vi "PH_HamamatsuCamera.panel.vi"(0 "object ref":refnum<vi>, 5 "error in (no error)":errorcluster) -> (19 "error out":errorcluster)   [LabVIEW 2014, in "PH_HamamatsuCamera.lvlib"]
doc: "This VI is the GUI to control a IEEE1394 Cam.\n\nLicense Agreement for this software:\n\nCopyright (C)\nGesellschaft für Schwerionenforschung, GSI\nPlanckstr. 1\n64291 Darmstadt\nGermany\n\nContact: D.Beck@gsi.de \n\nThis program is free software; you can redistribute it and/or modify it under the terms of the GNU General Public License as published by the Free Software Foundation; either version 2 of the license, or (at your option) any later version.\n\nThis program is distributed in the hope that it will be useful, but WITHOUT ANYW ARRANTY; without even the implied warranty of MERCHANTABILITY or FITNESS FOR A PARTICULAR PURPOSE. See the GNU General License for more details (http://www.gnu.org).\n\nGesellschaft für Schwerionenforschung, GSI\nPlanckstr. 1, 64291 Darmstadt, Germany\nFor all questions and ideas contact: M.Richter@gsi.de, H.Brand@gsi.de or D.Beck@gsi.de.\nLast update: 18-DEC-2002"
uses:
  PH_HamamatsuCamera.lvlib
  PH_StatusHandler/PH_StatusHandler.GUI element.ctl
  PH_HamamatsuCamera.ROI.ctl
  PH_HamamatsuCamera.Trigger Parameter.ctl
  PH_HamamatsuCamera.Parameter Set.ctl
  PH_HamamatsuCamera.Cam Parameter.ctl
  PH_Cam_BaseClass/PH_Cam_BaseClass.GUI Refs.ctl
  CSCore/CSObj/CSObj.lvlib
  CSCore/CSSystem/CSSystemLib/CSSystemLib.lvlib
  PH_Common/PH_Common.lvlib
  PH_Cam_BaseClass/PH_Cam_BaseClass.lvlib
  PH_Class/PH_Class.lvlib
  PH_StatusHandler/PH_StatusHandler.lvlib
panel:
  in  "Driver Original Polarity":u32(ring)=1 items=["Negative"=1, "Positive"=2]
  in  "Driver Original Mode":u32(ring)=1 items=["Internal"=1, "External Edge"=2, "External Level"=4, "Software"=32, "Fast Repetition"=64, "TDI"=128, "Trigger Start"=512, "Sync Readout"=1024]
  out "PSDB Status":u32(colorbox)=6618880 caption="PSDB"
  out "Status":T1 caption="Camera"
  in  "Tab Control":T2(tab)
  in  "Trigger Timeout":u32=1000 caption="ms"
  in  "Gain":dbl
  in  "Brightness":dbl
  in  "Shutter":dbl caption="s"
  in  "Start Cam":bool
  in  "Get Histogram":bool
  in  "Logarithmic":bool
  out "Histogram":u32[](graph)
  in  "Trigger Polarity":u32(ring) items=["No Info"]
  in  "Trigger Mode":u32(ring) items=["No Info"]
  in  "Save Image":bool
  in  "Show Image":bool
  in  "Palette":i32(ring) items=["Grey", "Binary", "Gradient", "Rainbow", "Temperature", "HMH"]
  in  "Scale Factor":i32=50 caption="%" min=30 max=500
  in  "Center of Gravity":bool
  in  "Subtract Background":bool
  in  "Center Cross":bool
  in  "Set ROI to Maximum":bool
  in  "ROI":T3
  out "Camera Details":T4
  out "Cam Error":errorcluster
  in  "Cam List":u32(ring)
  out "Frames per second":dbl(knob) scale=0.0..30.0 scale format="%.1f"
  in  "Get Frame Rate":bool
  in  "Parameter to set":T5=4212128 items=["SENSOR MODE"=4212128, "CCD MODE"=4212384, "READOUT MODE"=4211872, "ACTIVE VIEW INDEX"=4343136, "BITS PER CHANNEL"=4342976, "IMAGE PIXEL TYPE"=4343296, "BINNING"=4215968, "EXPOSURE TIME"=2049184, "CONTRAST GAIN"=3163312, "CONTRAST OFFSET"=3163328, "LIGHT MODE"=2114720, "SENSITIVITY"=2114992, "PHOTON IMAGING MODE"=2115200, "HIGH DYNAMIC RANGE MODE"=3163360, "WHITE BALANCE"=3163568, "TEMPERATURE"=2115232, "TEMPERATURE TARGET"=2115264, "SENSOR COOLER FAN"=2115296, "LINEBUNDLE HEIGHT"=4212192, "MECHANICAL SHUTTER"=2115488, "BACK FOCUS POSITION"=8422304, "TRIGGER CONNECTOR"=1066432, "TRIGGER SOURCE"=1066144, "OUTPUT TRIGGER SOURCE"=1852576, "TRIGGER GLOBAL EXPOSURE"=2049680, "FIRST TRIGGER BEHAVIOR"=2049696, "CHANNEL SYNC"=1852352, "READOUT DIRECTION"=4211904, "PRE HSYNC COUNT"=1852704, "INTERNAL LINE SPEED"=4191408, "INTERNAL LINE INTERVAL"=4191424]
  in  "Set Cam Parameter":bool caption="Set"
  in  "Value to set":dbl caption="Value"
  out "Parameters":T6[](array[typedef])
  in  "Trigger Parameters":T7={"Mode"=1, "Polarity"=1, "Times"=1, "Delay"=0.0} {"Polarity" items=["Negative"=1, "Positive"=2]; "Mode" items=["Internal"=1, "External Edge"=2, "External Level"=4, "Software"=32, "Fast Repetition"=64, "TDI"=128, "Trigger Start"=512, "Sync Readout"=1024]}
  in  "Delete":bool
  in  "Exit":bool
  # "PCS"
  # "3.40"
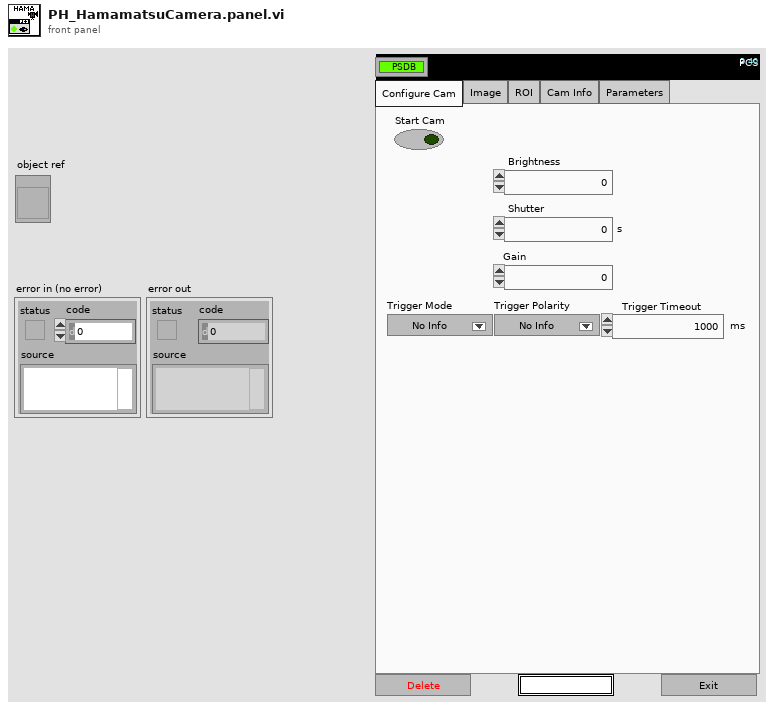
[diagram p1: front panel]
types:
  T1 = typedef "PH_StatusHandler.lvlib/PH_StatusHandler.GUI element.ctl" = u16
  T2 = enum32{"Configure Cam", "Image", "ROI", "Cam Info", "Parameters"}
  T3 = typedef "PH_HamamatsuCamera.lvlib/PH_HamamatsuCamera.ROI.ctl" = cluster{"Horizontal Offset":i32, "Vertical Offset":i32, "Horizontal Width":i32, "Vertical Width":i32}
  T4 = cluster{"Model":string, "Camera ID":string, "Firmware":string}
  T5 = typedef "PH_HamamatsuCamera.lvlib/PH_HamamatsuCamera.Cam Parameter.ctl" = u32
  T6 = typedef "PH_HamamatsuCamera.lvlib/PH_HamamatsuCamera.Parameter Set.ctl" = cluster{"Parameter":string, "Value":dbl, "Writable":bool, "Range":cluster{"min":dbl, "max":dbl, "step":dbl}, "Default":dbl, "Value Names":cluster{"Name":string, "Value":dbl}[], "Text Values":bool}
  T7 = typedef "PH_HamamatsuCamera.lvlib/PH_HamamatsuCamera.Trigger Parameter.ctl" = cluster{"Mode":u32, "Polarity":u32, "Times":u32, "Delay":dbl}
  T8 = typedef "PH_Cam_BaseClass.lvlib/PH_Cam_BaseClass.GUI Refs.ctl" = cluster{"Frame Rate":refnum<vi>, "Get Frame Rate":refnum<vi>, "Show Image":refnum<vi>, "Get Histogram":refnum<vi>, "Mapping":refnum<vi>, "Histogram":refnum<vi>, "Center Cross":refnum<vi>, "Center of Gravity":refnum<vi>, "Scale Factor [%]":refnum<vi>, "Save Image":refnum<vi>, "Palette":refnum<vi>, "Subtract Background":refnum<vi>, "Cam Error":refnum<vi>, "On":refnum<vi>, "Cam List":refnum<vi>}
  T9 = cluster{"Cam Base ClassGui Refs":T8, "PSDB Status":refnum<vi>, "Status":refnum<vi>}
  T10 = typedef "PH_HamamatsuCamera.lvlib/PH_HamamatsuCamera.i attribute.ctl" = cluster{"Gui Refs":cluster{"Camera Details":refnum<vi>, "ROI":refnum<vi>, "Set ROI to Maximum":refnum<vi>, "Trigger Parameters":refnum<vi>, "Brightness":refnum<vi>, "Shutter":refnum<vi>, "Gain":refnum<vi>, "Trigger Timeout":refnum<vi>, "Trigger Polarity":refnum<vi>, "Trigger Mode":refnum<vi>, "Parameters":refnum<vi>, "Set Cam Parameter":refnum<vi>, "Parameter to set":refnum<vi>, "Value to set":refnum<vi>}, "Cam":cluster{"Handle":i32, "Details":cluster{"Model":string, "Camera ID":string, "Firmware":string}, "Buffer Info":cluster{"height":u32, "width":u32, "datatype":u32}}, "H Offset":cluster{"Value":i32, "Minimum":i32, "Maximum":i32, "Increment":i32}, "V Offset":cluster{"Value":i32, "Minimum":i32, "Maximum":i32, "Increment":i32}, "H Width":cluster{"Value":i32, "Minimum":i32, "Maximum":i32, "Increment":i32}, "V Width":cluster{"Value":i32, "Minimum":i32, "Maximum":i32, "Increment":i32}, "Trigger Parameters":T7, "Trigger Timeout":u32, "Parameters":T6[], "Indicees Cam Parameters":cluster{"Brightness":i32, "Shutter":i32, "Gain":i32}, "Wanted Values":cluster{"Trigger Settings":T7[], "ROI":T3[], "Parameter":cluster{"Name":string, "Value":dbl}[]}}
  T11 = typedef "LVStringsAndValuesArrayTypeDef_U32.ctl" = cluster{"String":string, "Value":u32}[]
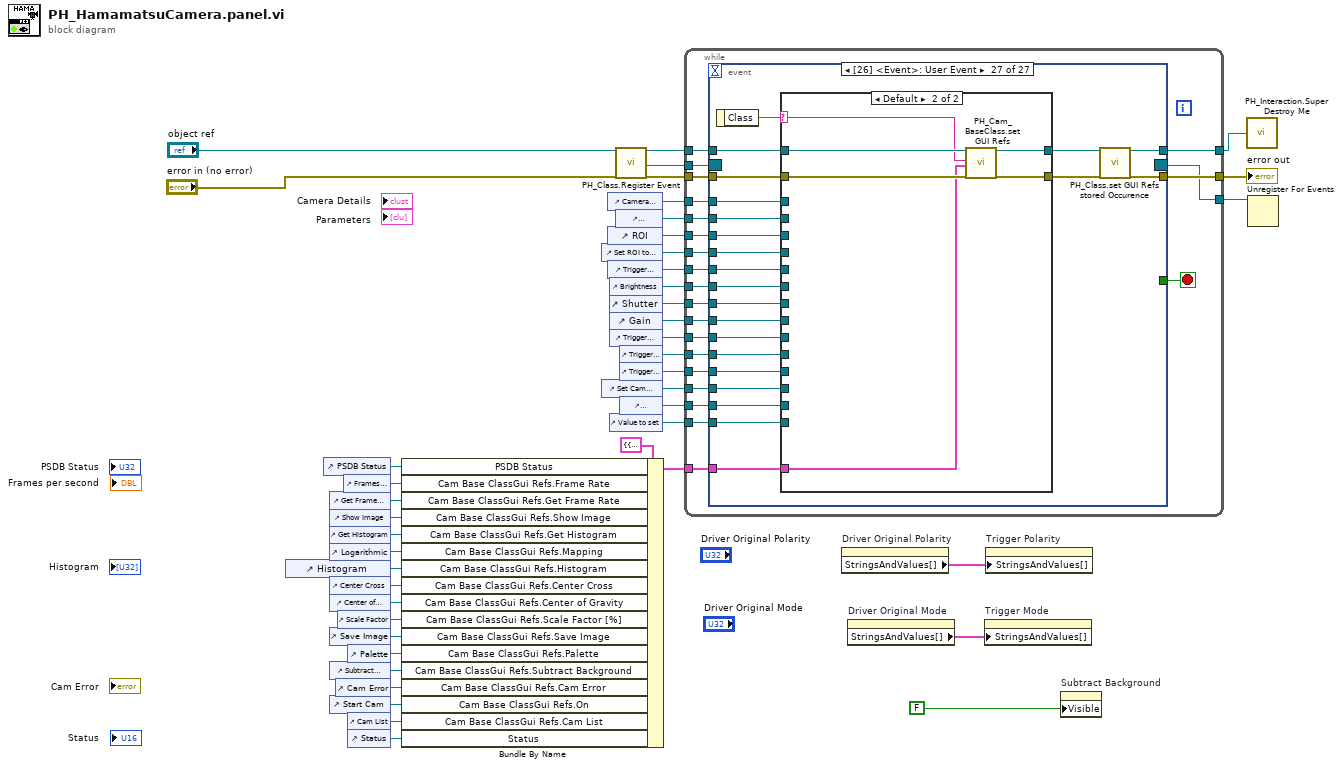
[diagram p0: block diagram]
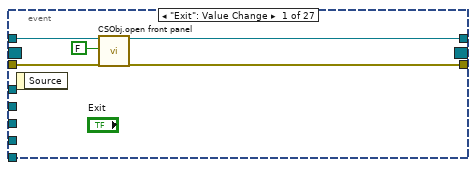
[diagram p2: hidden frame]
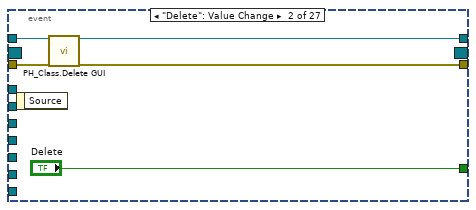
[diagram p3: hidden frame]
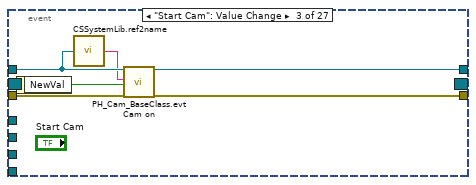
[diagram p4: hidden frame]
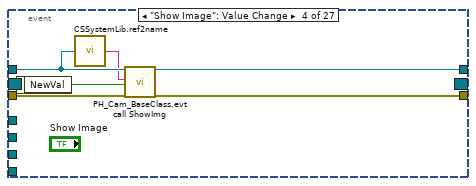
[diagram p5: hidden frame]
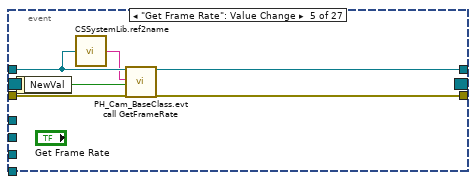
[diagram p6: hidden frame]
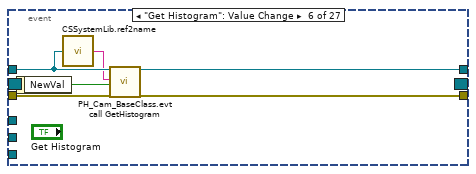
[diagram p7: hidden frame]
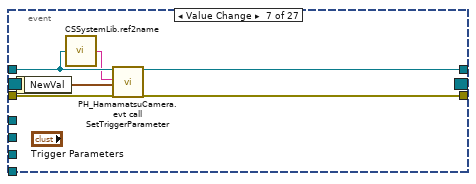
[diagram p8: hidden frame]
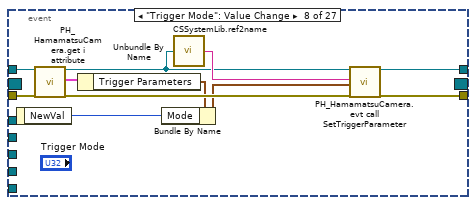
[diagram p9: hidden frame]
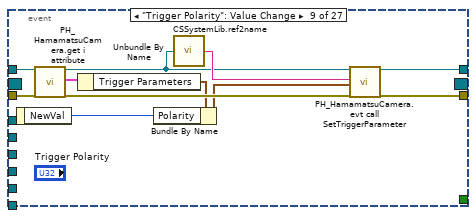
[diagram p10: hidden frame]
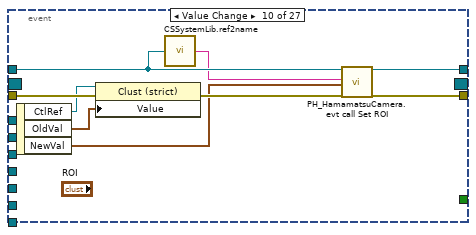
[diagram p11: hidden frame]
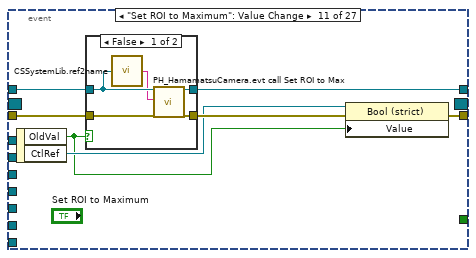
[diagram p12: hidden frame]
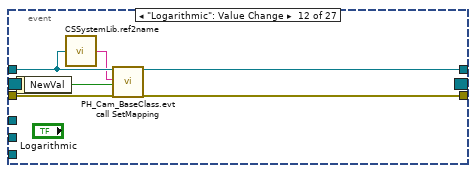
[diagram p14: hidden frame]
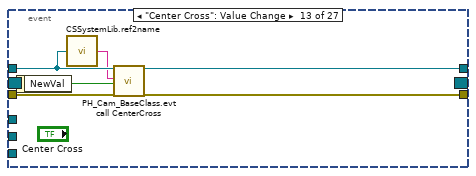
[diagram p15: hidden frame]
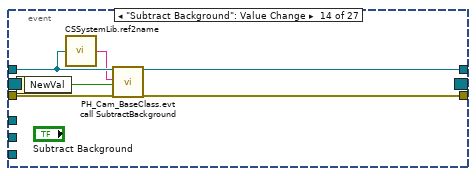
[diagram p16: hidden frame]
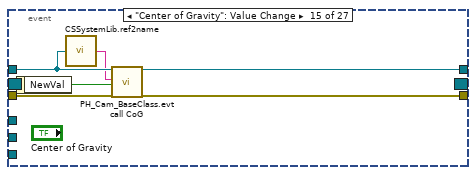
[diagram p17: hidden frame]
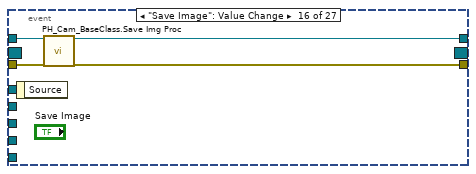
[diagram p18: hidden frame]
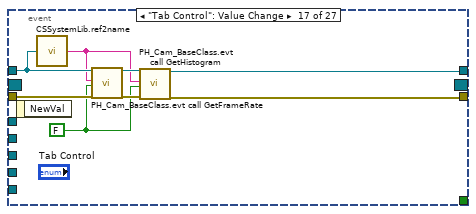
[diagram p19: hidden frame]
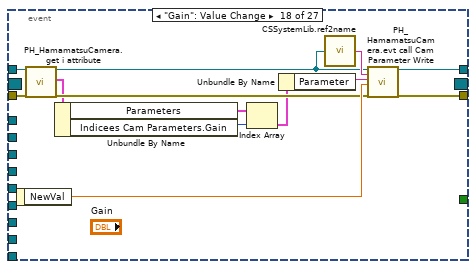
[diagram p20: hidden frame]
diagram:
  n1 = control-ref of="Histogram"() -> (w35:refnum<vi>)
  n2 = control-ref of="PSDB Status"() -> (w20:refnum<vi>)
  n3 = control-ref of="Get Frame Rate"() -> (w39:refnum<vi>)
  n4 = control-ref of="Show Image"() -> (w38:refnum<vi>)
  n5 = control-ref of="Get Histogram"() -> (w37:refnum<vi>)
  n6 = control-ref of="Logarithmic"() -> (w36:refnum<vi>)
  n7 = control-ref of="Center Cross"() -> (w34:refnum<vi>)
  n8 = control-ref of="Center of Gravity"() -> (w33:refnum<vi>)
  n9 = control-ref of="Save Image"() -> (w31:refnum<vi>)
  n10 = control-ref of="Subtract Background"() -> (w29:refnum<vi>)
  n11 = control-ref of="Start Cam"() -> (w26:refnum<vi>)
  n12 = control-ref of="Cam Error"() -> (w27:refnum<vi>)
  n13 = control-ref of="Scale Factor"() -> (w32:refnum<vi>)
  n14 = control-ref of="Frames per second"() -> (w40:refnum<vi>)
  n15 = control-ref of="Palette"() -> (w30:refnum<vi>)
  n16 = control-ref of="Cam List"() -> (w25:refnum<vi>)
  n17 = control-ref of="Status"() -> (w1:refnum<vi>)
  n18 = Bundle By Name(cluster=T9 {"Cam Base ClassGui Refs"={"Frame Rate"=refnum, "Get Frame Rate"=refnum, "Show Image"=refnum, "Get Histogram"=refnum, "Mapping"=refnum, "Histogram"=refnum, "Center Cross"=refnum, "Center of Gravity"=refnum, "Scale Factor [%]"=refnum, "Save Image"=refnum, "Palette"=refnum, "Subtract Background"=refnum, "Cam Error"=refnum, "On"=refnum, "Cam List"=refnum}, "PSDB Status"=refnum, "Status"=refnum} ("GUI Refs to set"), "PSDB Status"=w20, "Cam Base ClassGui Refs.Frame Rate"=w40, "Cam Base ClassGui Refs.Get Frame Rate"=w39, "Cam Base ClassGui Refs.Show Image"=w38, "Cam Base ClassGui Refs.Get Histogram"=w37, "Cam Base ClassGui Refs.Mapping"=w36, "Cam Base ClassGui Refs.Histogram"=w35, "Cam Base ClassGui Refs.Center Cross"=w34, "Cam Base ClassGui Refs.Center of Gravity"=w33, "Cam Base ClassGui Refs.Scale Factor [%]"=w32, "Cam Base ClassGui Refs.Save Image"=w31, "Cam Base ClassGui Refs.Palette"=w30, "Cam Base ClassGui Refs.Subtract Background"=w29, "Cam Base ClassGui Refs.Cam Error"=w27, "Cam Base ClassGui Refs.On"=w26, "Cam Base ClassGui Refs.Cam List"=w25, "Status"=w1) -> (w19:T9)
  n19 = control-ref of="Set ROI to Maximum"() -> (w15:refnum<vi>)
  n20 = control-ref of="Set Cam Parameter"() -> (w7:refnum<vi>)
  n21 = control-ref of="Camera Details"() -> (w18:refnum<vi>)
  n22 = control-ref of="ROI"() -> (w16:refnum<vi>)
  n23 = control-ref of="Trigger Parameters"() -> (w14:refnum<vi>)
  n24 = control-ref of="Brightness"() -> (w13:refnum<vi>)
  n25 = control-ref of="Shutter"() -> (w12:refnum<vi>)
  n26 = control-ref of="Gain"() -> (w11:refnum<vi>)
  n27 = control-ref of="Trigger Timeout"() -> (w10:refnum<vi>)
  n28 = control-ref of="Value to set"() -> (w5:refnum<vi>)
  n29 = call "PH_Class.Register Event.vi"("i ref in"="object ref", "error in (no error)"="error in (no error)") -> ("i ref out"=w24:refnum<vi>, "Event Registration Refnum"=w22:refnum<event-registration>, "error out"=w23:errorcluster)  [unwired: 15 in]
  n30 = control-ref of="Parameters"() -> (w17:refnum<vi>)
  n31 = control-ref of="Trigger Polarity"() -> (w9:refnum<vi>)
  n32 = control-ref of="Trigger Mode"() -> (w8:refnum<vi>)
  n33 = control-ref of="Parameter to set"() -> (w6:refnum<vi>)
  n34 = while {
    tunnel: w24 -> [w63]
    tunnel: [w62] -> w43
    tunnel: w23 -> [w65]
    tunnel: [w64] -> w44
    tunnel: w22 -> [w61]
    tunnel: [w60] -> w21
    tunnel: w19 -> [w59]
    tunnel: w18 -> [w58]
    tunnel: w17 -> [w57]
    tunnel: w16 -> [w56]
    tunnel: w15 -> [w55]
    tunnel: w14 -> [w54]
    tunnel: w13 -> [w53]
    tunnel: w12 -> [w52]
    tunnel: w11 -> [w51]
    tunnel: w10 -> [w50]
    tunnel: w9 -> [w49]
    tunnel: w8 -> [w48]
    tunnel: w7 -> [w47]
    tunnel: w6 -> [w46]
    tunnel: w5 -> [w45]
    stop <- w66 stop-if-true
    n35 = event shown="[26] <Event>: User Event" {
      selector: w61 -> [_ _ _ _ _ _ _ _ _ _ _ _ _ _ _ _ _ _ _ _ _ _ _ _ _ _ _]
      dyn-events: [_ _ _ _ _ _ _ _ _ _ _ _ _ _ _ _ _ _ _ _ _ _ _ _ _ _ _] -> w60
      timeout: _ -> [_ _ _ _ _ _ _ _ _ _ _ _ _ _ _ _ _ _ _ _ _ _ _ _ _ _ _]
      tunnel: [_ "Delete" _ _ _ _ _ _ _ _ _ _ _ _ _ _ _ _ _ _ _ _ _ _ _ _ _] -> w66
      tunnel: w63 -> [w71 w74 w79 w85 w91 w97 w103 w112 w123 w135 w141 w154 w160 w166 w172 w178 w182 w194 w207 w220 w229 w235 w243 w254 w264 w269 w293]
      tunnel: w65 -> [w69 w75 w82 w88 w94 w100 w106 w117 w128 w131 w144 w157 w163 w169 w175 w179 w185 w200 w213 w226 w232 w238 w246 w248 w262 w271 w292]
      tunnel: [w68 w72 w81 w87 w93 w99 w105 w116 w127 w137 w140 w156 w162 w168 w174 w176 w183 w198 w211 w224 w230 w236 w244 w255 w265 w270 w287] -> w64
      tunnel: [w67 w73 w80 w86 w92 w98 w104 w115 w126 w136 w142 w155 w161 w167 w173 w177 w186 w199 w212 w225 w231 w237 w245 w256 w266 w268 w289] -> w62
      tunnel: w59 -> [_ _ _ _ _ _ _ _ _ _ _ _ _ _ _ _ _ _ _ _ _ _ _ _ _ _ w290]
      tunnel: w58 -> [_ _ _ _ _ _ _ _ _ _ _ _ _ _ _ _ _ _ _ _ _ _ _ _ _ _ w285]
      tunnel: w57 -> [_ _ _ _ _ _ _ _ _ _ _ _ _ _ _ _ _ _ _ _ _ _ _ _ _ _ w284]
      tunnel: w56 -> [_ _ _ _ _ _ _ _ _ _ _ _ _ _ _ _ _ _ _ _ _ _ _ _ _ _ w283]
      tunnel: w55 -> [_ _ _ _ _ _ _ _ _ _ _ _ _ _ _ _ _ _ _ _ _ _ _ _ _ _ w282]
      tunnel: w54 -> [_ _ _ _ _ _ _ _ _ _ _ _ _ _ _ _ _ _ _ _ _ _ _ _ _ _ w281]
      tunnel: w53 -> [_ _ _ _ _ _ _ _ _ _ _ _ _ _ _ _ _ _ _ _ _ _ _ _ _ _ w280]
      tunnel: w52 -> [_ _ _ _ _ _ _ _ _ _ _ _ _ _ _ _ _ _ _ _ _ _ _ _ _ _ w279]
      tunnel: w51 -> [_ _ _ _ _ _ _ _ _ _ _ _ _ _ _ _ _ _ _ _ _ _ _ _ _ _ w278]
      tunnel: w50 -> [_ _ _ _ _ _ _ _ _ _ _ _ _ _ _ _ _ _ _ _ _ _ _ _ _ _ w277]
      tunnel: w49 -> [_ _ _ _ _ _ _ _ _ _ _ _ _ _ _ _ _ _ _ _ _ _ _ _ _ _ w276]
      tunnel: w48 -> [_ _ _ _ _ _ _ _ _ _ _ _ _ _ _ _ _ _ _ _ _ _ _ _ _ _ w275]
      tunnel: w47 -> [_ _ _ _ _ _ _ _ _ _ _ _ _ _ _ _ _ _ _ _ _ _ _ _ _ _ w274]
      tunnel: w46 -> [_ _ _ _ _ _ _ _ _ _ _ _ _ _ _ _ _ _ _ _ _ _ _ _ _ _ w273]
      tunnel: w45 -> [_ _ _ _ _ _ _ _ _ _ _ _ _ _ _ _ _ _ _ _ _ _ _ _ _ _ w272]
      event "Exit": Value Change {
        n36 = event-data() -> ()  [unwired: 1 in, 1 out]
        n37 = call "CSObj.open front panel.vi"("i ref in"=w71, "frontPanelOpen"=FALSE ("front panel open"), "error in (no error)"=w69) -> ("i ref out"=w67:refnum<vi>, "error out"=w68:errorcluster)  [unwired: 15 in]
      }
      event "Delete": Value Change {
        n38 = event-data() -> ()  [unwired: 1 in, 1 out]
        n39 = call "PH_Class.Delete GUI.vi"("VI in"=w74, "error in (no error)"=w75) -> ("VI out"=w73:refnum<vi>, "error out"=w72:errorcluster)  [unwired: 16 in]
      }
      event "Start Cam": Value Change {
        n40 = event-data() -> ("NewVal"=w77:bool)  [unwired: 1 in]
        n41 = call "CSSystemLib.ref2name.vi"("obj refnum"=w79) -> ("name"=w78:string)
        n42 = call "PH_Cam_BaseClass.evt Cam on.vi"("i ref in"=w79, "Instance"=w78, "Cam on"=w77, "error in (no error)"=w82) -> ("i ref out"=w80:refnum<vi>, "error out"=w81:errorcluster)  [unwired: 14 in]
      }
      event "Show Image": Value Change {
        n43 = event-data() -> ("NewVal"=w83:bool)  [unwired: 1 in]
        n44 = call "CSSystemLib.ref2name.vi"("obj refnum"=w85) -> ("name"=w84:string)
        n45 = call "PH_Cam_BaseClass.evt call ShowImg.vi"("i ref in"=w85, "Instance"=w84, "Start Cam"=w83, "error in (no error)"=w88) -> ("i ref out"=w86:refnum<vi>, "error out"=w87:errorcluster)  [unwired: 14 in]
      }
      event "Get Frame Rate": Value Change {
        n46 = event-data() -> ("NewVal"=w89:bool)  [unwired: 1 in]
        n47 = call "CSSystemLib.ref2name.vi"("obj refnum"=w91) -> ("name"=w90:string)
        n48 = call "PH_Cam_BaseClass.evt call GetFrameRate.vi"("i ref in"=w91, "Instance"=w90, "Get Frame Rate"=w89, "error in (no error)"=w94) -> ("i ref out"=w92:refnum<vi>, "error out"=w93:errorcluster)  [unwired: 14 in]
      }
      event "Get Histogram": Value Change {
        n49 = event-data() -> ("NewVal"=w95:bool)  [unwired: 1 in]
        n50 = call "CSSystemLib.ref2name.vi"("obj refnum"=w97) -> ("name"=w96:string)
        n51 = call "PH_Cam_BaseClass.evt call GetHistogram.vi"("i ref in"=w97, "Instance"=w96, "Get Histogram"=w95, "error in (no error)"=w100) -> ("i ref out"=w98:refnum<vi>, "error out"=w99:errorcluster)  [unwired: 14 in]
      }
      event Value Change {
        n52 = event-data() -> ("NewVal"=w101:T7)  [unwired: 1 in]
        n53 = call "CSSystemLib.ref2name.vi"("obj refnum"=w103) -> ("name"=w102:string)
        n54 = call "PH_HamamatsuCamera.evt call SetTriggerParameter.vi"("i ref in"=w103, "Instance"=w102, "Trigger Parameters"=w101, "error in (no error)"=w106) -> ("i ref out"=w104:refnum<vi>, "error out"=w105:errorcluster)  [unwired: 14 in]
      }
      event "Trigger Mode": Value Change {
        n55 = event-data() -> ("NewVal"=w107:u32)  [unwired: 1 in]
        n56 = call "PH_HamamatsuCamera.get i attribute.vi"("i ref in"=w112, "error in (no error)"=w117) -> ("i ref out"=w111:refnum<vi>, "i attribute"=w110:T10, "error out"=w113:errorcluster)  [unwired: 15 in]
        n57 = Unbundle By Name(w110) -> ("Trigger Parameters"=w109:T7)
        n58 = Bundle By Name(cluster=w109, "Mode"=w107) -> (w108:T7)
        n59 = call "CSSystemLib.ref2name.vi"("obj refnum"=w111) -> ("name"=w114:string)
        n60 = call "PH_HamamatsuCamera.evt call SetTriggerParameter.vi"("i ref in"=w111, "Instance"=w114, "Trigger Parameters"=w108, "error in (no error)"=w113) -> ("i ref out"=w115:refnum<vi>, "error out"=w116:errorcluster)  [unwired: 14 in]
      }
      event "Trigger Polarity": Value Change {
        n61 = event-data() -> ("NewVal"=w118:u32)  [unwired: 1 in]
        n62 = call "PH_HamamatsuCamera.get i attribute.vi"("i ref in"=w123, "error in (no error)"=w128) -> ("i ref out"=w122:refnum<vi>, "i attribute"=w121:T10, "error out"=w124:errorcluster)  [unwired: 15 in]
        n63 = Unbundle By Name(w121) -> ("Trigger Parameters"=w120:T7)
        n64 = Bundle By Name(cluster=w120, "Polarity"=w118) -> (w119:T7)
        n65 = call "CSSystemLib.ref2name.vi"("obj refnum"=w122) -> ("name"=w125:string)
        n66 = call "PH_HamamatsuCamera.evt call SetTriggerParameter.vi"("i ref in"=w122, "Instance"=w125, "Trigger Parameters"=w119, "error in (no error)"=w124) -> ("i ref out"=w126:refnum<vi>, "error out"=w127:errorcluster)  [unwired: 14 in]
      }
      event Value Change {
        n67 = event-data() -> ("CtlRef"=w130:refnum<vi>, "OldVal"=w132:T3, "NewVal"=w129:T3)  [unwired: 1 in]
        n68 = property class="Clust (strict)"(reference=w130, error in=w131, "Value"=w132) -> (error out=w133:errorcluster)  [unwired: 1 out]
        n69 = call "CSSystemLib.ref2name.vi"("obj refnum"=w135) -> ("name"=w134:string)
        n70 = call "PH_HamamatsuCamera.evt call Set ROI.vi"("i ref in"=w135, "Instance"=w134, "ROI"=w129, "error in (no error)"=w133) -> ("i ref out"=w136:refnum<vi>, "error out"=w137:errorcluster)  [unwired: 14 in]
      }
      event "Set ROI to Maximum": Value Change {
        n71 = event-data() -> ("OldVal"=w138:bool, "CtlRef"=w139:refnum<vi>)  [unwired: 1 in]
        n72 = case shown="False" w138 {
          tunnel: w144 -> [w149 w150]
          tunnel: [w148 w150] -> w143
          tunnel: [w147 w151] -> w142
          tunnel: w141 -> [w146 w151]
          frame False {
            n73 = call "CSSystemLib.ref2name.vi"("obj refnum"=w146) -> ("name"=w145:string)
            n74 = call "PH_HamamatsuCamera.evt call Set ROI to Max.vi"("i ref in"=w146, "Instance"=w145, "error in (no error)"=w149) -> ("i ref out"=w147:refnum<vi>, "error out"=w148:errorcluster)  [unwired: 15 in]
          }
          frame True {
          }
        }
        n75 = property class="Bool (strict)"(reference=w139, error in=w143, "Value"=w138) -> (error out=w140:errorcluster)  [unwired: 1 out]
      }
      event "Logarithmic": Value Change {
        n76 = event-data() -> ("NewVal"=w152:bool)  [unwired: 1 in]
        n77 = call "CSSystemLib.ref2name.vi"("obj refnum"=w154) -> ("name"=w153:string)
        n78 = call "PH_Cam_BaseClass.evt call SetMapping.vi"("i ref in"=w154, "Instance"=w153, "Get Histogram"=w152, "error in (no error)"=w157) -> ("i ref out"=w155:refnum<vi>, "error out"=w156:errorcluster)  [unwired: 14 in]
      }
      event "Center Cross": Value Change {
        n79 = event-data() -> ("NewVal"=w158:bool)  [unwired: 1 in]
        n80 = call "CSSystemLib.ref2name.vi"("obj refnum"=w160) -> ("name"=w159:string)
        n81 = call "PH_Cam_BaseClass.evt call CenterCross.vi"("i ref in"=w160, "Instance"=w159, "Center Cross"=w158, "error in (no error)"=w163) -> ("i ref out"=w161:refnum<vi>, "error out"=w162:errorcluster)  [unwired: 14 in]
      }
      event "Subtract Background": Value Change {
        n82 = event-data() -> ("NewVal"=w164:bool)  [unwired: 1 in]
        n83 = call "CSSystemLib.ref2name.vi"("obj refnum"=w166) -> ("name"=w165:string)
        n84 = call "PH_Cam_BaseClass.evt call SubtractBackground.vi"("i ref in"=w166, "Instance"=w165, "Subtract Background"=w164, "error in (no error)"=w169) -> ("i ref out"=w167:refnum<vi>, "error out"=w168:errorcluster)  [unwired: 14 in]
      }
      event "Center of Gravity": Value Change {
        n85 = event-data() -> ("NewVal"=w170:bool)  [unwired: 1 in]
        n86 = call "CSSystemLib.ref2name.vi"("obj refnum"=w172) -> ("name"=w171:string)
        n87 = call "PH_Cam_BaseClass.evt call CoG.vi"("i ref in"=w172, "Instance"=w171, "Set CoG"=w170, "error in (no error)"=w175) -> ("i ref out"=w173:refnum<vi>, "error out"=w174:errorcluster)  [unwired: 14 in]
      }
      event "Save Image": Value Change {
        n88 = event-data() -> ()  [unwired: 1 in, 1 out]
        n89 = call "PH_Cam_BaseClass.Save Img Proc.vi"("VI in"=w178, "error in (no error)"=w179) -> ("VI out"=w177:refnum<vi>, "error out"=w176:errorcluster)  [unwired: 16 in]
      }
      event "Tab Control": Value Change {
        w180 = FALSE
        n90 = event-data() -> ()  [unwired: 1 in, 1 out]
        n91 = call "CSSystemLib.ref2name.vi"("obj refnum"=w182) -> ("name"=w181:string)
        n92 = call "PH_Cam_BaseClass.evt call GetFrameRate.vi"("i ref in"=w182, "Instance"=w181, "Get Frame Rate"=w180, "error in (no error)"=w185) -> ("i ref out"=w187:refnum<vi>, "error out"=w184:errorcluster)  [unwired: 14 in]
        n93 = call "PH_Cam_BaseClass.evt call GetHistogram.vi"("i ref in"=w187, "Instance"=w181, "Get Histogram"=w180, "error in (no error)"=w184) -> ("i ref out"=w186:refnum<vi>, "error out"=w183:errorcluster)  [unwired: 14 in]
      }
      event "Gain": Value Change {
        n94 = event-data() -> ("NewVal"=w196:dbl)  [unwired: 1 in]
        n95 = call "PH_HamamatsuCamera.get i attribute.vi"("i ref in"=w194, "error in (no error)"=w200) -> ("i ref out"=w193:refnum<vi>, "i attribute"=w192:T10, "error out"=w195:errorcluster)  [unwired: 15 in]
        n96 = Unbundle By Name(w192) -> ("Parameters"=w191:T6[], "Indicees Cam Parameters.Gain"=w190:i32)
        n97 = Index Array(array=w191, index=w190) -> (element=w189:T6)
        n98 = Unbundle By Name(w189) -> ("Parameter"=w188:string)
        n99 = call "CSSystemLib.ref2name.vi"("obj refnum"=w193) -> ("name"=w197:string)
        n100 = call "PH_HamamatsuCamera.evt call Cam Parameter Write.vi"("i ref in"=w193, "Instance"=w197, "Parameter to set"=w188, "Value"=w196, "error in (no error)"=w195) -> ("i ref out"=w199:refnum<vi>, "error out"=w198:errorcluster)  [unwired: 13 in]
      }
      event "Brightness": Value Change {
        n101 = event-data() -> ("NewVal"=w209:dbl)  [unwired: 1 in]
        n102 = call "PH_HamamatsuCamera.get i attribute.vi"("i ref in"=w207, "error in (no error)"=w213) -> ("i ref out"=w206:refnum<vi>, "i attribute"=w202:T10, "error out"=w208:errorcluster)  [unwired: 15 in]
        n103 = Unbundle By Name(w202) -> ("Parameters"=w205:T6[], "Indicees Cam Parameters.Brightness"=w204:i32)
        n104 = Index Array(array=w205, index=w204) -> (element=w203:T6)
        n105 = Unbundle By Name(w203) -> ("Parameter"=w201:string)
        n106 = call "CSSystemLib.ref2name.vi"("obj refnum"=w206) -> ("name"=w210:string)
        n107 = call "PH_HamamatsuCamera.evt call Cam Parameter Write.vi"("i ref in"=w206, "Instance"=w210, "Parameter to set"=w201, "Value"=w209, "error in (no error)"=w208) -> ("i ref out"=w212:refnum<vi>, "error out"=w211:errorcluster)  [unwired: 13 in]
      }
      event "Shutter": Value Change {
        n108 = event-data() -> ("NewVal"=w222:dbl)  [unwired: 1 in]
        n109 = call "PH_HamamatsuCamera.get i attribute.vi"("i ref in"=w220, "error in (no error)"=w226) -> ("i ref out"=w219:refnum<vi>, "i attribute"=w215:T10, "error out"=w221:errorcluster)  [unwired: 15 in]
        n110 = Unbundle By Name(w215) -> ("Parameters"=w218:T6[], "Indicees Cam Parameters.Shutter"=w217:i32)
        n111 = Index Array(array=w218, index=w217) -> (element=w216:T6)
        n112 = Unbundle By Name(w216) -> ("Parameter"=w214:string)
        n113 = call "CSSystemLib.ref2name.vi"("obj refnum"=w219) -> ("name"=w223:string)
        n114 = call "PH_HamamatsuCamera.evt call Cam Parameter Write.vi"("i ref in"=w219, "Instance"=w223, "Parameter to set"=w214, "Value"=w222, "error in (no error)"=w221) -> ("i ref out"=w225:refnum<vi>, "error out"=w224:errorcluster)  [unwired: 13 in]
      }
      event "Trigger Timeout": Value Change {
        n115 = event-data() -> ("NewVal"=w227:u32)  [unwired: 1 in]
        n116 = call "CSSystemLib.ref2name.vi"("obj refnum"=w229) -> ("name"=w228:string)
        n117 = call "PH_HamamatsuCamera.evt call SetTimeout.vi"("i ref in"=w229, "Instance"=w228, "TO [ms]"=w227, "error in (no error)"=w232) -> ("i ref out"=w231:refnum<vi>, "error out"=w230:errorcluster)  [unwired: 14 in]
      }
      event "Palette": Value Change {
        n118 = event-data() -> ("NewVal"=w233:i32)  [unwired: 1 in]
        n119 = call "CSSystemLib.ref2name.vi"("obj refnum"=w235) -> ("name"=w234:string)
        n120 = call "PH_Cam_BaseClass.evt call SetPalette.vi"("i ref in"=w235, "Instance"=w234, "Palette"=w233, "error in (no error)"=w238) -> ("i ref out"=w237:refnum<vi>, "error out"=w236:errorcluster)  [unwired: 14 in]
      }
      event "Scale Factor": Value Change {
        n121 = event-data() -> ("NewVal"=w240:i32)  [unwired: 1 in]
        n122 = call "CSSystemLib.ref2name.vi"("obj refnum"=w243) -> ("name"=w242:string)
        n123 = Divide(x=w240, y=100) -> (x/y=w239:dbl)
        n124 = call "PH_Cam_BaseClass.evt call SetScaleFactor.vi"("i ref in"=w243, "Instance"=w242, "Scale Factor [%]"=w239, "error in (no error)"=w246) -> ("i ref out"=w245:refnum<vi>, "error out"=w244:errorcluster)  [unwired: 14 in]
      }
      event "Cam List": Value Change {
        n125 = event-data() -> ("CtlRef"=w252:refnum<vi>)  [unwired: 1 in]
        n126 = property class="Ring (strict)"(reference=w252, error in=w248) -> (error out=w247:errorcluster, "Strings []"=w250:string[], "Value"=w251:u32)  [unwired: 1 out]
        n127 = call "CSSystemLib.ref2name.vi"("obj refnum"=w254) -> ("name"=w253:string)
        n128 = Index Array(array=w250, index=w251) -> (element=w249:string)
        n129 = call "PH_Cam_BaseClass.evt call Connect.vi"("i ref in"=w254, "Instance"=w253, "Cam Name"=w249, "error in (no error)"=w247) -> ("i ref out"=w256:refnum<vi>, "error out"=w255:errorcluster)  [unwired: 14 in]
      }
      event "Set Cam Parameter": Value Change {
        n130 = event-data() -> ()  [unwired: 1 in, 1 out]
        n131 = property on="Parameter to set" class="Ring (strict)"(error in=w262) -> (error out=w259:errorcluster, "Strings []"=w261:string[], "Value"=w260:u32)  [unwired: 1 in, 1 out]
        n132 = Index Array(array=w261, index=w260) -> (element=w258:string)
        n133 = call "CSSystemLib.ref2name.vi"("obj refnum"=w264) -> ("name"=w263:string)
        n134 = call "PH_HamamatsuCamera.evt call Cam Parameter Write.vi"("i ref in"=w264, "Instance"=w263, "Parameter to set"=w258, "Value"="Value to set", "error in (no error)"=w259) -> ("i ref out"=w266:refnum<vi>, "error out"=w265:errorcluster)  [unwired: 13 in]
      }
      event Value Change {
        n135 = event-data() -> ()  [unwired: 1 in, 1 out]
        n136 = call "PH_HamamatsuCamera.set Visibility of Cam Attribute Value Set Knobs.vi"("VI in"=w269, "Parameter"="Parameter to set", "error in (no error)"=w271) -> ("VI out"=w268:refnum<vi>, "error out"=w270:errorcluster)  [unwired: 15 in]
      }
      event User Event {
        n137 = event-data() -> ("Class"=w291:string)  [unwired: 1 in]
        n138 = case shown="Default" w291 {
          selector: w291 -> [_ w318]
          tunnel: w293 -> [w311 w322]
          tunnel: w292 -> [w309 w321]
          tunnel: [w310 w320] -> w288
          tunnel: [w308 w319] -> w286
          tunnel: w290 -> [_ w317]
          tunnel: w285 -> [w307 _]
          tunnel: w284 -> [w306 _]
          tunnel: w283 -> [w305 _]
          tunnel: w282 -> [w304 _]
          tunnel: w281 -> [w303 _]
          tunnel: w280 -> [w302 _]
          tunnel: w279 -> [w301 _]
          tunnel: w278 -> [w300 _]
          tunnel: w277 -> [w299 _]
          tunnel: w276 -> [w298 _]
          tunnel: w275 -> [w297 _]
          tunnel: w274 -> [w296 _]
          tunnel: w273 -> [w295 _]
          tunnel: w272 -> [w294 _]
          frame "PH_HamamatsuCamera" {
            n139 = call "PH_HamamatsuCamera.get data to modify.vi"("i ref in"=w311, "ms timeout (10000)"=-1, "error in (no error)"=w309) -> ("i ref out"=w316:refnum<vi>, "i attribute"=w313:T10, "error out"=w315:errorcluster)  [unwired: 13 in, 1 out]
            n140 = Bundle By Name(cluster=w313, "Gui Refs.Camera Details"=w307, "Gui Refs.Parameters"=w306, "Gui Refs.ROI"=w305, "Gui Refs.Set ROI to Maximum"=w304, "Gui Refs.Trigger Parameters"=w303, "Gui Refs.Brightness"=w302, "Gui Refs.Shutter"=w301, "Gui Refs.Gain"=w300, "Gui Refs.Trigger Timeout"=w299, "Gui Refs.Trigger Polarity"=w298, "Gui Refs.Trigger Mode"=w297, "Gui Refs.Set Cam Parameter"=w296, "Gui Refs.Parameter to set"=w295, "Gui Refs.Value to set"=w294) -> (w312:T10)
            n141 = call "PH_HamamatsuCamera.set modified data.vi"("i ref in"=w316, "i attribute"=w312, "error in (no error)"=w315) -> ("i ref out"=w310:refnum<vi>, "error out"=w308:errorcluster)  [unwired: 15 in]
          }
          frame Default {
            n142 = call "PH_Cam_BaseClass.set GUI Refs.vi"("VI in"=w322, "Class"=w318, "GUI Refs to set"=w317, "error in (no error)"=w321) -> ("VI out"=w320:refnum<vi>, "error out"=w319:errorcluster)  [unwired: 14 in]
          }
        }
        n143 = call "PH_Class.set GUI Refs stored Occurence.vi"("i ref in"=w288, "error in (no error)"=w286) -> ("i ref out"=w289:refnum<vi>, "error out"=w287:errorcluster)  [unwired: 16 in]
      }
    }
  }
  "error out" <- w44
  n144 = property on="Driver Original Polarity" class="Ring (strict)"() -> ("StringsAndValues[]"=w42:T11)  [unwired: 2 in, 2 out]
  n145 = property on="Driver Original Mode" class="Ring (strict)"() -> ("StringsAndValues[]"=w41:T11)  [unwired: 2 in, 2 out]
  n146 = property on="Trigger Mode" class="Ring (strict)"("StringsAndValues[]"=w41) -> ()  [unwired: 2 in, 2 out]
  n147 = property on="Trigger Polarity" class="Ring (strict)"("StringsAndValues[]"=w42) -> ()  [unwired: 2 in, 2 out]
  n148 = property on="Subtract Background" class="Bool (strict)"("Visible"=FALSE) -> ()  [unwired: 2 in, 2 out]
  n149 = call "PH_Interaction.Super Destroy Me.vi"("i ref out"=w43) -> ()
  n150 = Unregister For Events(event registration refnum=w21) -> ()  [unwired: 1 in, 1 out]
